vi "Tag Get__icon_lib_labview_project_api.vi"(8 "error in (no error)":errorcluster, 10 "Tag Name":string, 11 "Build Spec Reference":refnum<vi>) -> (0 "error out":errorcluster, 1 "Value":variant, 3 "Build Spec Reference Dup":refnum<vi>, 4 "Is Persistent":bool)   [LabVIEW 2016, in "LabVIEW Project API__icon_lib_labview_project_api.lvlib"]
doc: "Gets a Project Tag's Value\n\n<b>Author:</b> JG\n\n<b>ICON Technologies Pty Ltd</b>\nCopyright (C) 1990-2009\nAll Rights Reserved"
uses:
  LabVIEW Project API__icon_lib_labview_project_api.lvlib
panel:
  # "Output"
  # "Input"
  # "ICON Technologies Pty Ltd\nCopyright (C) 1990-2009\nAll Rights Reserved"
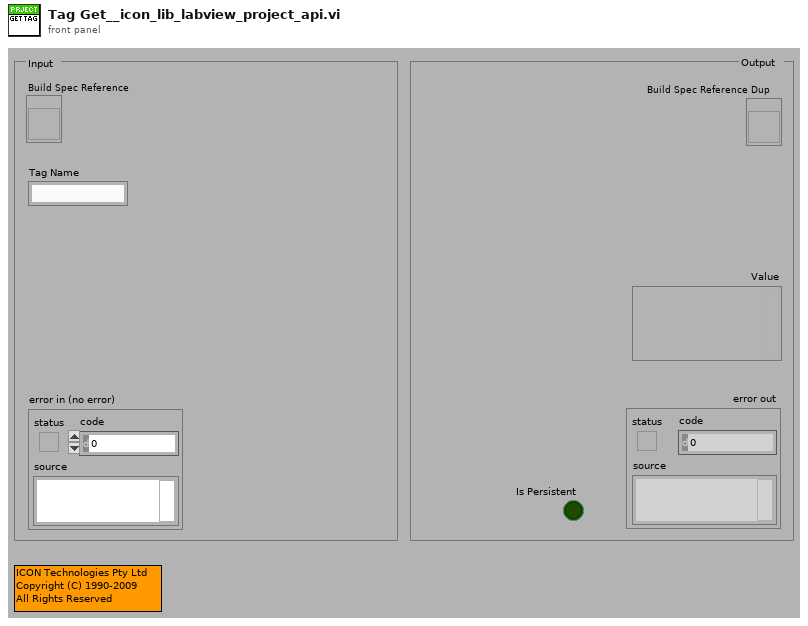
[diagram p1: front panel]
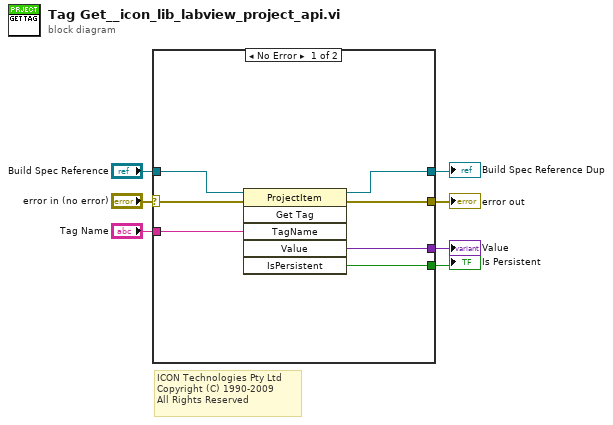
[diagram p0: block diagram]
diagram:
  # "ICON Technologies Pty Ltd\nCopyright (C) 1990-2009\nAll Rights Reserved"
  n1 = case shown="No Error" "error in (no error)" {
    selector: "error in (no error)" -> [w13 w16]
    tunnel: [w9 w16] -> w6
    tunnel: "Build Spec Reference" -> [w14 w15]
    tunnel: [w12 w15] -> w4
    tunnel: [w10 _] -> w3
    tunnel: "Tag Name" -> [w11 _]
    tunnel: [w8 _] -> w1
    frame No Error {
      n2 = invoke class="ProjectItem" method="Get Tag"(reference=w14, error in=w13, "TagName"=w11) -> (reference out=w12:refnum<vi>, error out=w9:errorcluster, "Value"=w10:variant, "IsPersistent"=w8:bool)  [unwired: 3 in, 2 out]
    }
    frame Error {
    }
  }
  "error out" <- w6
  "Build Spec Reference Dup" <- w4
  "Value" <- w3
  "Is Persistent" <- w1
